vi "LEP_RV_StartLaunch.vi"(8 "error in (no error)":errorcluster) -> (0 "error out":errorcluster)   [LabVIEW 2011]
doc: "Download and execute built VxWorks downloadable module and attach the LabVIEW Embedded debuger."
uses:
  LEP_RV_Commands.ctl
  LEP_RV_Config.ctl
  <vilib>/Platform/EmbProject/utilities/Emb_Utility_AppAction.ctl
  <vilib>/LabVIEW Targets/Embedded/ASWServer/MPU_ASWServer_GeneralIcons.ctl
  <vilib>/LabVIEW Targets/Embedded/ASWServer/MPU_ASWServer_GeneralCtrls.ctl
  LEP_RV_LaunchGlobals.vi
  <vilib>/Platform/EmbProject/Plugins/utilities/LEP_Utilities_GetInfoGlobals.vi
  <vilib>/Instr/_visa.llb/VISA Configure Serial Port (Instr).vi
panel:
  in  "Client installed":bool
  in  "Remember password":bool
  in  "Password":string
  in  "User name":string
  in  "Compiler server name":string
  in  "Connect to a network compile server":bool
  in  "buildSpec ID":string
  in  "error string":string
  in  "Error Indicator":bool[](array[boolean])
  in  "Node ID List":i32[](array[numeric])
  in  "Message List":string[][](array[string])
  in  "Active File Count":i32
  in  "embeddedSessionID":u32
  in  "subtarget":string
  in  "path":path
  in  "preallocate UI Enabled":bool
  in  "target display name":string
  in  "SourceFiles":path[](array[path])
  in  "ExternalFiles":path[](array[path])
  in  "ProjectPath":path
  in  "display name":string
  in  "typeID":string
  in  "debug occurrence":refnum<k4>
  in  "Item ID":string
  in  "Root ID":string
  in  "target ID":u32
  in  "build ID":u32
  in  "MaxElements":u32
  in  "DebugSerialPort":string
  in  "DebugSerialBaud":u32
  in  "Context":refnum<vi>
  in  "UpdateClusters":u32
  in  "UpdateArrays":u32
  in  "Update":u32
  in  "BreakpointsConfig":cluster{"Clear on Start":bool}
  in  "File List":path[](array[path])
  in  "action":T1
  in  "Config":T2={"Enable debugging"=FALSE, "Debug Options"=0, "Use stack variables"=FALSE, "Generate serial only"=FALSE, "Generate guard code"=FALSE, "Generate Integer Only"=FALSE, "Generate C Function Calls"=TRUE, "ExpressionFolding"=TRUE, "Constant Allocation"=0, "Constant Deallocation"=0, "Build Specification ID"="", "Preprocessor symbols (define)"="", "Compiler Flags"="", "Linker Flags"="", "Mode"=1, "Optimization"=2, "Optimize for time"=FALSE, "Enable cross-module optimization"=FALSE, "Include paths"=[], "Optimize heap size"=TRUE, "Use MicroLib"=FALSE, "Debug Mode"=2, "Enable profile information"=FALSE, "Host name"="board", "Use DHCP"=TRUE, "IP address"="0.0.0.0", "Subnet mask"="", "Gateway"="0.0.0.0", "Primary DNS"="0.0.0.0", "Secondary DNS"="0.0.0.0", "MAC in target memory"=TRUE, "MAC address"="", "Console output"=1, "Target serial port"=1} {"Constant Deallocation" items=["Out of Scope", "VI End", "Application End"]; "Constant Allocation" items=["First Use", "Containing Loop", "VI Initialization", "Application Initialization"]; "Target serial port" items=["0", "1", "2", "3"]; "Console output" items=["Processor status window", "Serial port"]; "Optimization" items=["Level 0 (-O0)", "Level 1 (-O1)", "Level 2 (-O2)", "Level 3 (-O3)"]; "Mode" items=["ARM-Mode", "Thumb-Mode"]; "Debug Options" items=["Use ULINK Debugger", "Use Simulator"]; "Debug Mode" items=["Instrumented (serial port)", "Instrumented (TCP/IP)", "Non-instrumented (JTAG/USB)"]}
  in  "TopLevelVI":path
  in  "UV Project File":path
  in  "Target Name":string
  in  "Build Path":path
  in  "Commands":T3
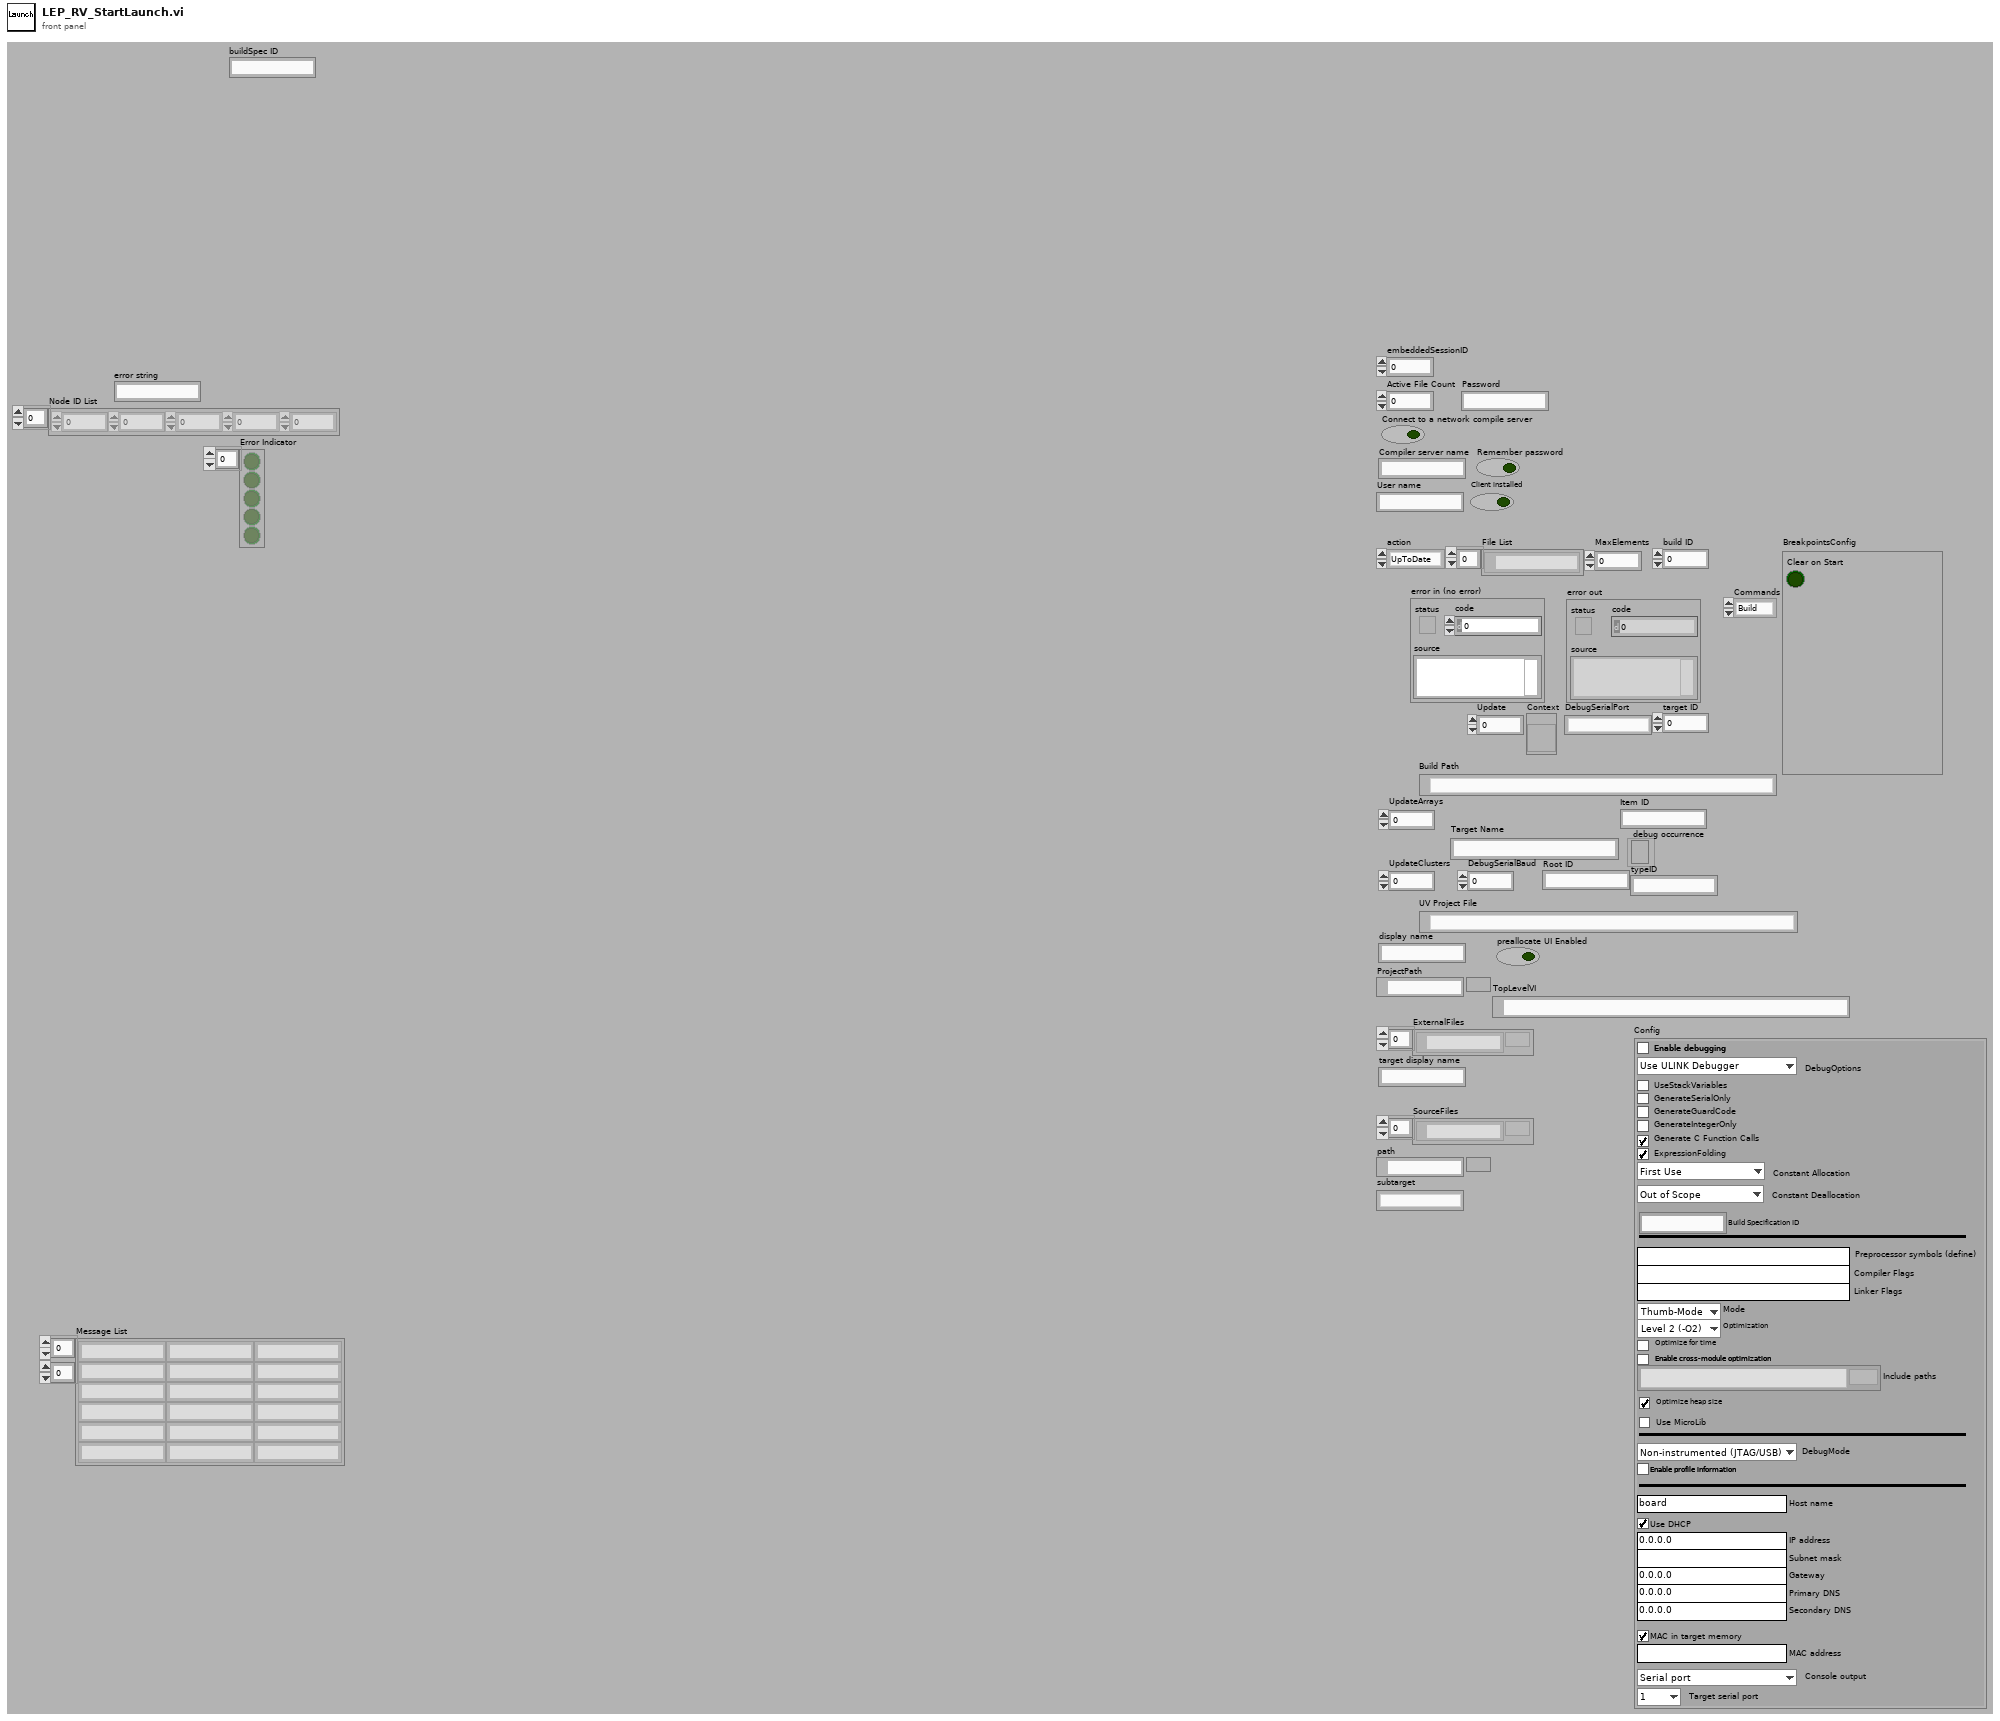
[diagram p1: front panel]
types:
  T1 = typedef "Emb_Utility_AppAction.ctl" = enum16{"UpToDate", "Build", "Cancel", "Error"}
  T2 = typedef "LEP_RV_Config.ctl" = cluster{"Enable debugging":bool, "Debug Options":u16, "Use stack variables":bool, "Generate serial only":bool, "Generate guard code":bool, "Generate Integer Only":bool, "Generate C Function Calls":bool, "ExpressionFolding":bool, "Constant Allocation":u16, "Constant Deallocation":u16, "Build Specification ID":string, "Preprocessor symbols (define)":string, "Compiler Flags":string, "Linker Flags":string, "Mode":u16, "Optimization":u16, "Optimize for time":bool, "Enable cross-module optimization":bool, "Include paths":path[], "Optimize heap size":bool, "Use MicroLib":bool, "Debug Mode":u16, "Enable profile information":bool, "Host name":string, "Use DHCP":bool, "IP address":string, "Subnet mask":string, "Gateway":string, "Primary DNS":string, "Secondary DNS":string, "MAC in target memory":bool, "MAC address":string, "Console output":u16, "Target serial port":u16}
  T3 = typedef "LEP_RV_Commands.ctl" = enum16{"Build", "Rebuild", "Run", "Debug", "Profile"}
  T4 = typedef "MPU_ASWServer_GeneralIcons.ctl" = enum16{"Complete", "Disconnected", "Error", "Initializing", "Ready", "Running", "Stopped", "Unknown", "No Change"}
  T5 = typedef "MPU_ASWServer_GeneralCtrls.ctl" = enum16{"Build Status", "Download Status", "Target Name", "Target Type", "Application Name"}
  T6 = enum16{"Build Successful", "Build Failed", "Build Cancelled"}
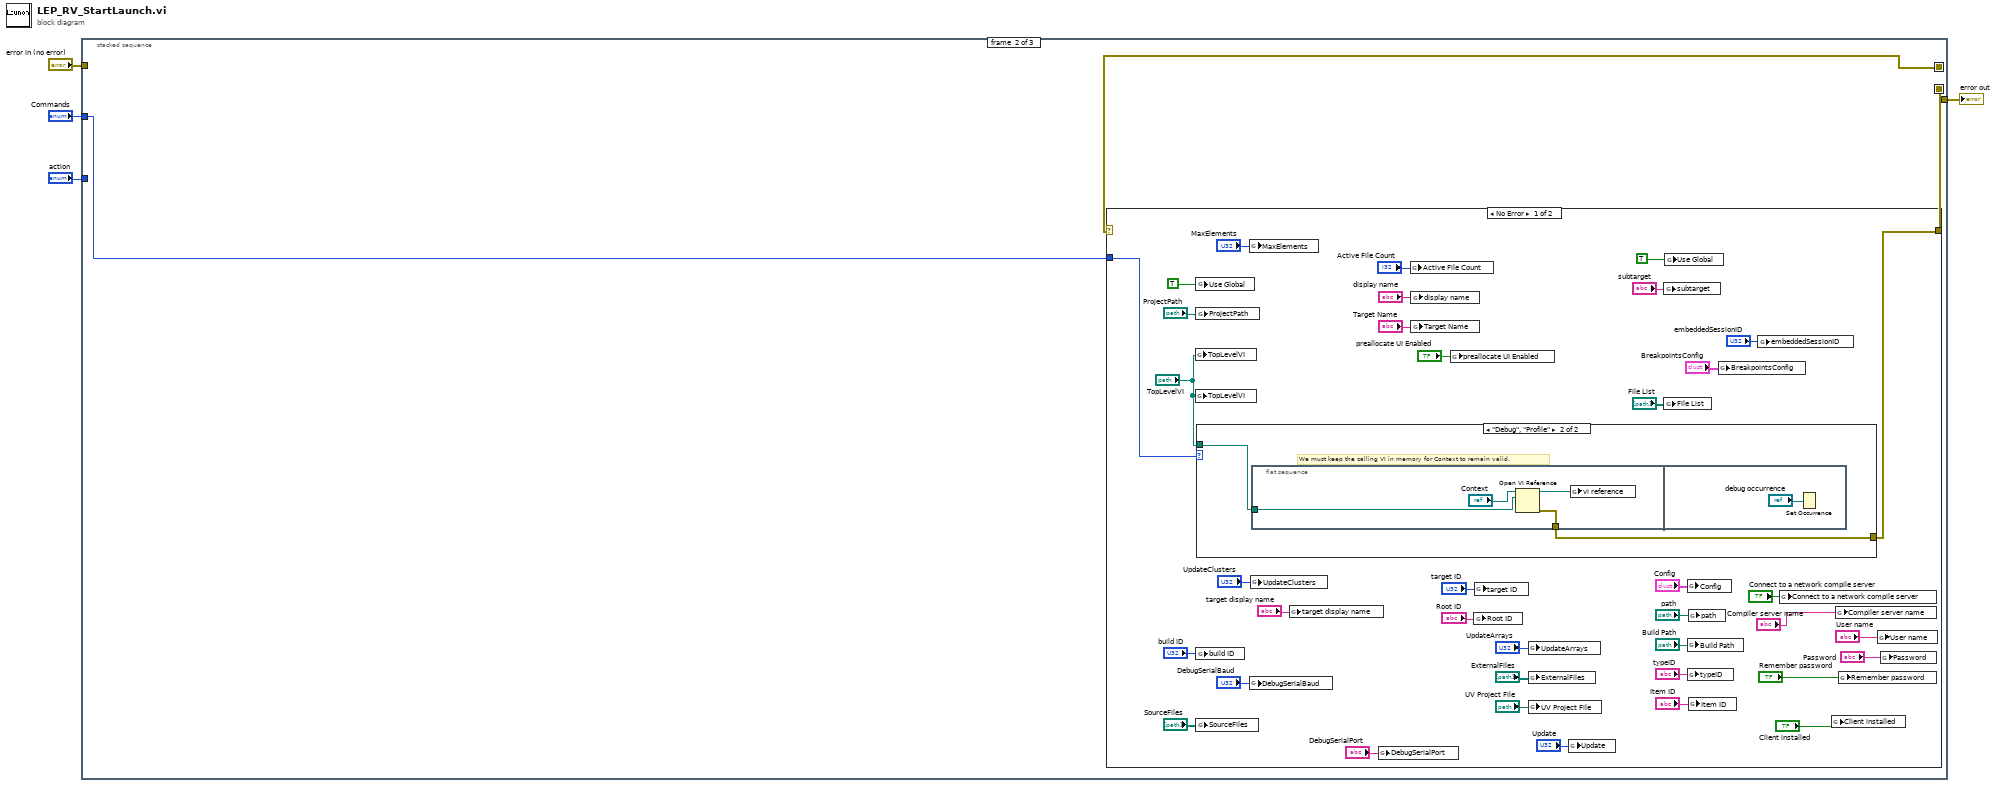
[diagram p0: block diagram]
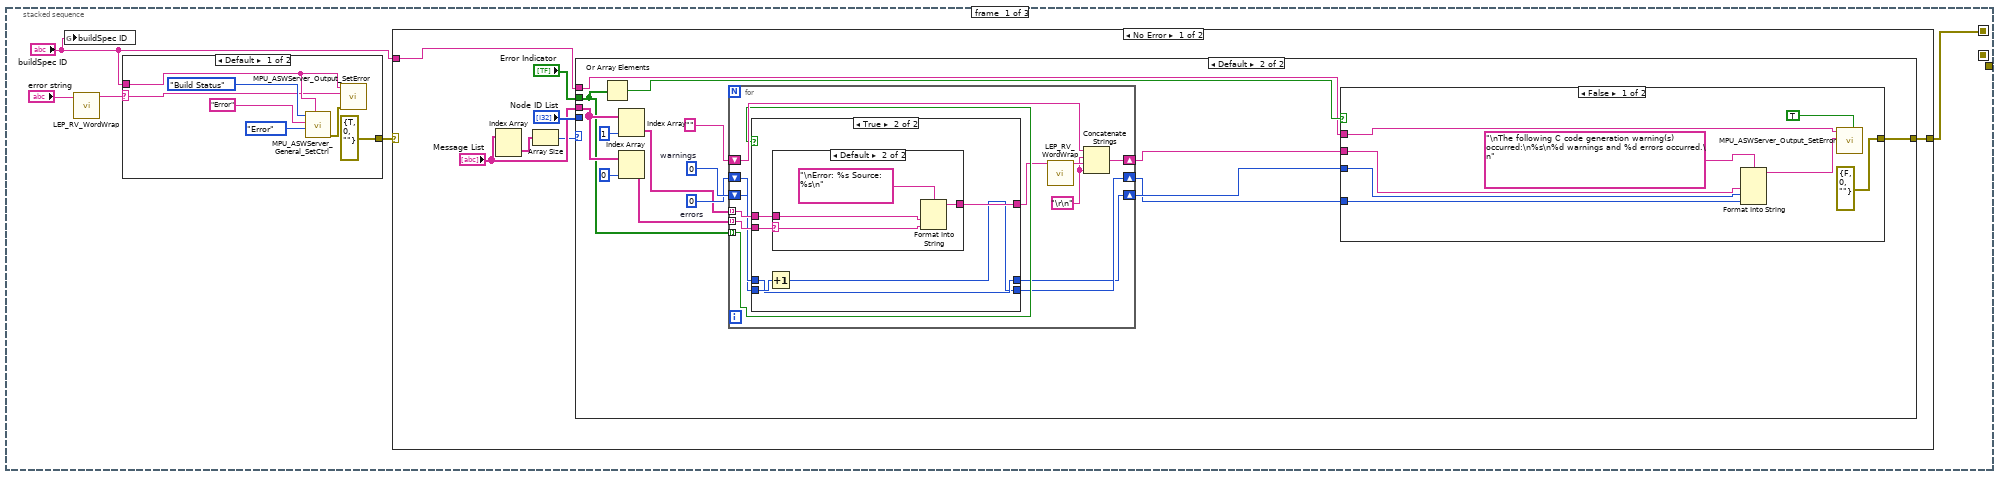
[diagram p2: hidden frame]
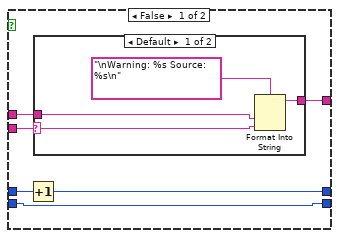
[diagram p4: hidden frame]
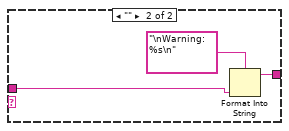
[diagram p5: hidden frame]
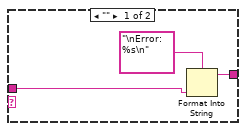
[diagram p6: hidden frame]
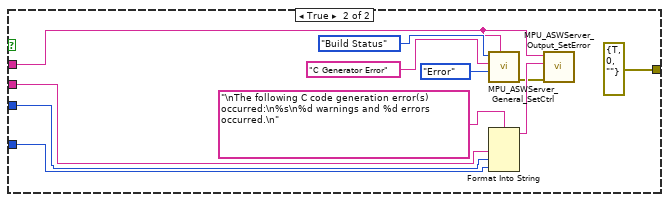
[diagram p7: hidden frame]
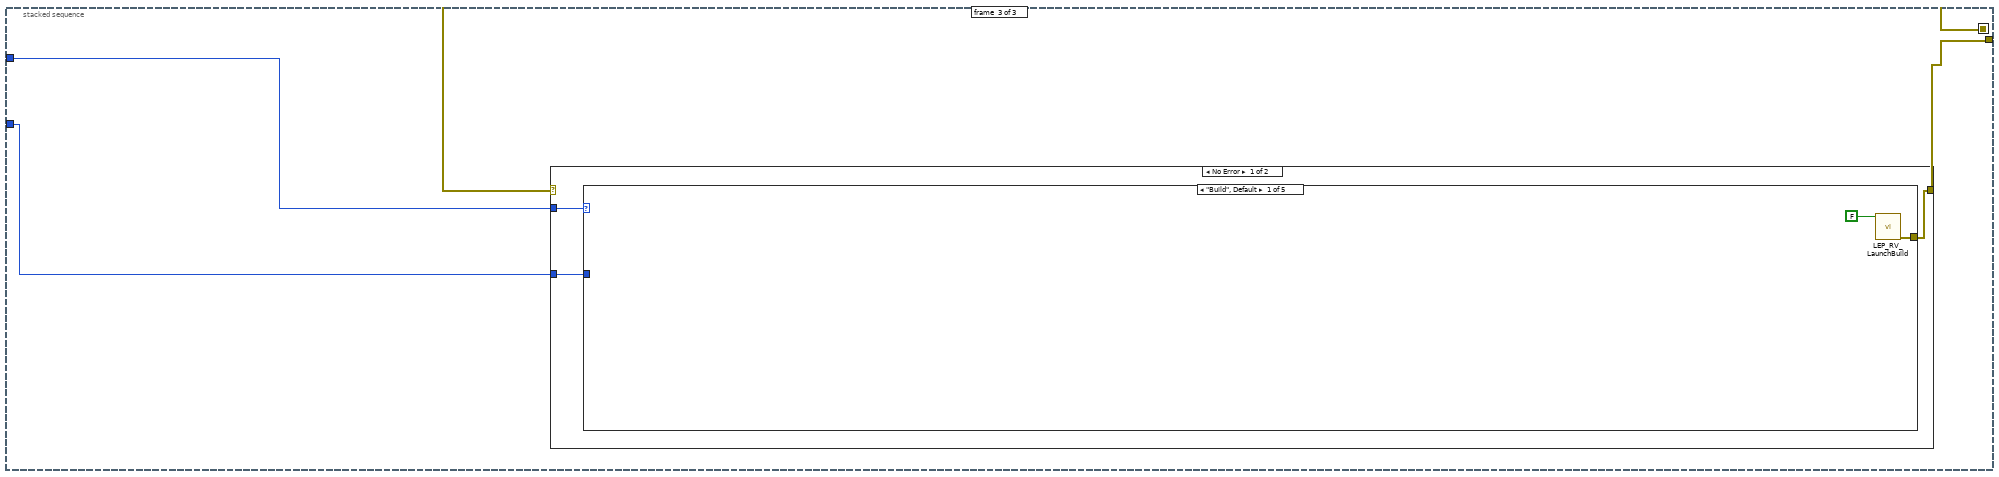
[diagram p12: hidden frame]
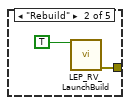
[diagram p13: hidden frame]
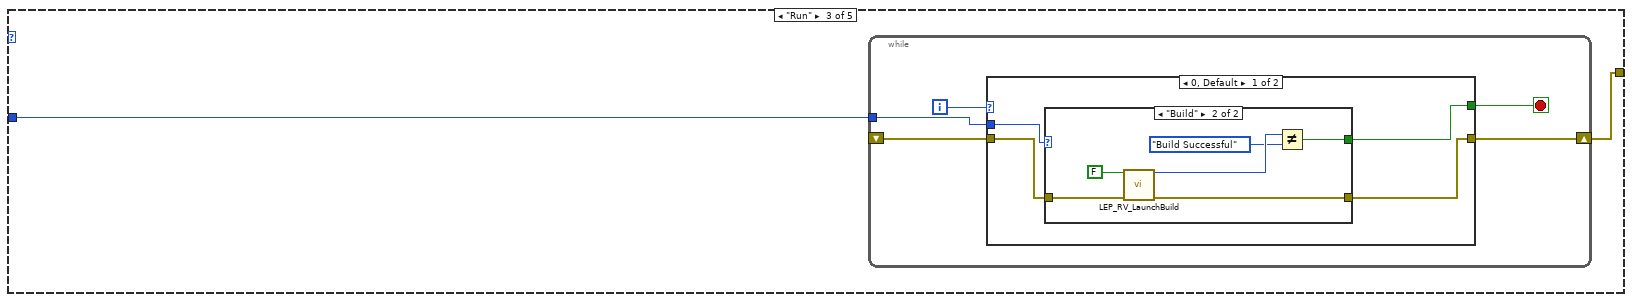
[diagram p14: hidden frame]
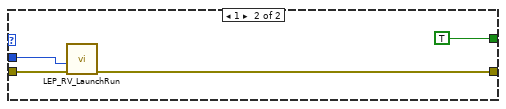
[diagram p16: hidden frame]
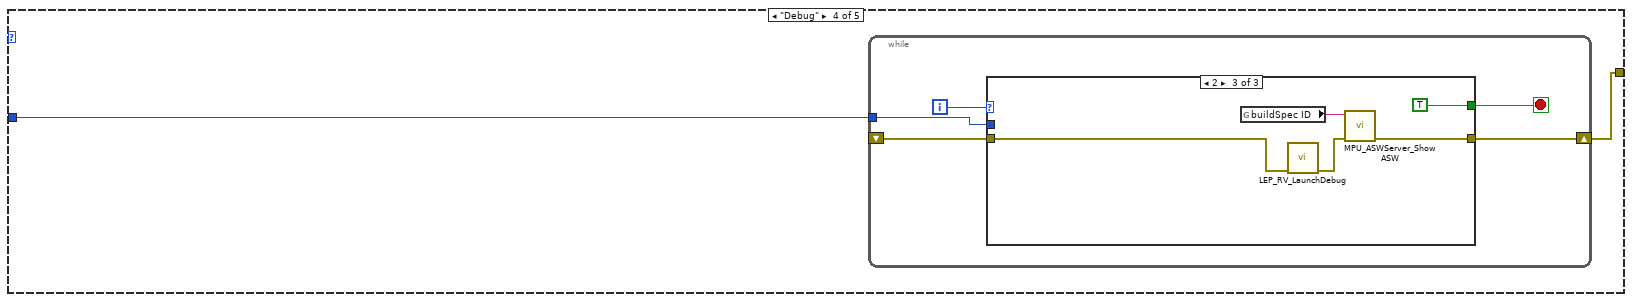
[diagram p17: hidden frame]
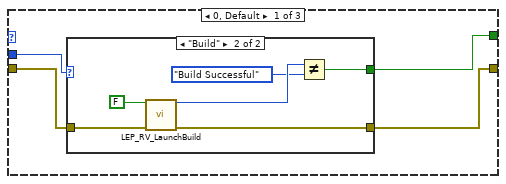
[diagram p18: hidden frame]
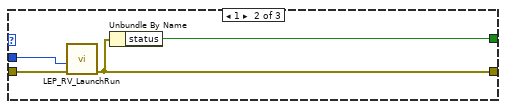
[diagram p20: hidden frame]
diagram:
  n1 = stacked-sequence {
    seq-local: [_ w98 _] -> [_ _ w146]
    seq-local: [w8 _ _] -> [_ w97 _]
    tunnel: "error in (no error)" -> [_ _ _]
    tunnel: [_ _ w149] -> w3
    tunnel: "Commands" -> [_ w99 w148]
    tunnel: "action" -> [_ _ w147]
    frame #0 {
      n2 = global write "LEP_RV_LaunchGlobals.vi" "buildSpec ID"("buildSpec ID") -> ()
      n3 = call "LEP_RV_WordWrap.vi"("input string"="error string") -> ("output string"=w5:string)  [unwired: 10 in]
      n4 = case shown="Default" w5 {
        selector: w5 -> [w92 _]
        tunnel: "buildSpec ID" -> [w96 _]
        tunnel: [errorcluster {"status"=TRUE, "code"=0, "source"=""} ("error out") _] -> w7
        frame Default {
          n5 = call <vilib>:"MPU_ASWServer_General_SetCtrl.vi"("buildSpec ID"=w96, "icon"=MPU_ASWServer_GeneralIcons."Error", "value"="Error", "control"=MPU_ASWServer_GeneralCtrls."Build Status") -> ("error out"=w91:errorcluster)  [unwired: 5 in, 2 out]
          n6 = call <vilib>:"MPU_ASWServer_Output_SetError.vi"("error in"=w91, "error str"=w92, "buildSpec ID"=w96) -> ()  [unwired: 2 in, 5 out]
        }
        frame "", "CGenErr" {
        }
      }
      n7 = case shown="No Error" w7 {
        selector: w7 -> [_ w89]
        tunnel: "buildSpec ID" -> [w14 _]
        tunnel: [w10 w89] -> w8
        frame No Error {
          n8 = Index Array(array="Message List") -> (element=w12:string[])  [unwired: 2 in]
          n9 = Array Size(array=w12) -> (size(s)=w11:i32)
          n10 = case shown="Default" w11 {
            tunnel: "Message List" -> [_ w23]
            tunnel: "Error Indicator" -> [_ w22]
            tunnel: "Node ID List" -> [_ _]
            tunnel: w14 -> [_ w21]
            tunnel: [_ w20] -> w10
            frame 0 {
            }
            frame Default {
              w29 = u32 0  # warnings
              w28 = u32 0  # errors
              n11 = Or Array Elements(Boolean array=w22) -> (logical OR=w24:bool)
              n12 = Index Array(array=w23, index (col)=1 ("index (row)")) -> (element=w26:string[])  [unwired: 1 in]
              n13 = Index Array(array=w23, index (col)=0 ("index (row)")) -> (element=w27:string[])  [unwired: 1 in]
              n14 = for {
                shift-right: [w42] -> w17
                shift-left: "" -> [w43]
                tunnel: w26 -> [w41] mode=indexing
                tunnel: w27 -> [w40] mode=indexing
                tunnel: w22 -> [w39] mode=indexing
                shift-right: [w36] -> w30
                shift-left: w28 -> [w37]
                shift-right: [w35] -> w31
                shift-left: w29 -> [w38]
                w32 = "\r\n"
                n15 = case shown="True" w39 {
                  tunnel: [w48 w62] -> w34
                  tunnel: w41 -> [w49 w61]
                  tunnel: w40 -> [w44 w57]
                  tunnel: w38 -> [w46 w59]
                  tunnel: w37 -> [w47 w60]
                  tunnel: [w47 w58] -> w36
                  tunnel: [w45 w59] -> w35
                  frame False {
                    n16 = Increment(x=w46) -> (x+1=w45:u32)
                    n17 = case shown="Default" w44 {
                      selector: w44 -> [w52 _]
                      tunnel: w49 -> [w51 w55]
                      tunnel: [w50 w54] -> w48
                      frame Default {
                        n18 = Format Into String(format string="\nWarning: %s Source: %s\n", w51, w52) -> (resulting string=w50:string)  [unwired: 2 in, 1 out]
                      }
                      frame "" {
                        n19 = Format Into String(format string="\nWarning: %s\n", w55) -> (resulting string=w54:string)  [unwired: 2 in, 1 out]
                      }
                    }
                  }
                  frame True {
                    n20 = Increment(x=w60) -> (x+1=w58:u32)
                    n21 = case shown="Default" w57 {
                      selector: w57 -> [_ w66]
                      tunnel: [w64 w68] -> w62
                      tunnel: w61 -> [w63 w67]
                      frame "" {
                        n22 = Format Into String(format string="\nError: %s\n", w63) -> (resulting string=w64:string)  [unwired: 2 in, 1 out]
                      }
                      frame Default {
                        n23 = Format Into String(format string="\nError: %s Source: %s\n", w67, w66) -> (resulting string=w68:string)  [unwired: 2 in, 1 out]
                      }
                    }
                  }
                }
                n24 = call "LEP_RV_WordWrap.vi"("input string"=w34) -> ("output string"=w33:string)  [unwired: 10 in]
                n25 = Concatenate Strings(w43, w32, w33, w32) -> (w42:string)
              }
              n26 = case shown="False" w24 {
                tunnel: w21 -> [w72 w81]
                tunnel: w30 -> [w73 w79]
                tunnel: w31 -> [w74 w78]
                tunnel: w17 -> [w75 w87]
                tunnel: [errorcluster {"status"=FALSE, "code"=0, "source"=""} ("error out") errorcluster {"status"=TRUE, "code"=0, "source"=""} ("error out")] -> w20
                frame False {
                  n27 = Format Into String(format string="\nThe following C code generation warning(s) occurred:\n%s\n%d warnings and %d errors occurred.\n", w75, w74, w73) -> (resulting string=w71:string)  [unwired: 2 in, 1 out]
                  n28 = call <vilib>:"MPU_ASWServer_Output_SetError.vi"("warning only (F)"=TRUE ("warning only"), "error str"=w71, "buildSpec ID"=w72) -> ()  [unwired: 2 in, 5 out]
                }
                frame True {
                  n29 = call <vilib>:"MPU_ASWServer_General_SetCtrl.vi"("buildSpec ID"=w81, "icon"=MPU_ASWServer_GeneralIcons."Error", "value"="C Generator Error", "control"=MPU_ASWServer_GeneralCtrls."Build Status") -> ("error out"=w82:errorcluster)  [unwired: 5 in, 2 out]
                  n30 = Format Into String(format string="\nThe following C code generation error(s) occurred:\n%s\n%d warnings and %d errors occurred.\n", w87, w78, w79) -> (resulting string=w86:string)  [unwired: 2 in, 1 out]
                  n31 = call <vilib>:"MPU_ASWServer_Output_SetError.vi"("error in"=w82, "error str"=w86, "buildSpec ID"=w81) -> ()  [unwired: 2 in, 5 out]
                }
              }
            }
          }
        }
        frame Error {
        }
      }
    }
    frame #1 {
      n32 = case shown="No Error" w97 {
        selector: w97 -> [_ w145]
        tunnel: w99 -> [w137 _]
        tunnel: [w136 w145] -> w98
        frame No Error {
          n33 = global write "LEP_RV_LaunchGlobals.vi" "TopLevelVI"("TopLevelVI") -> ()
          n34 = global write "LEP_Utilities_GetInfoGlobals.vi" "TopLevelVI"("TopLevelVI") -> ()
          n35 = global write "LEP_Utilities_GetInfoGlobals.vi" "Use Global"(TRUE ("Use Global")) -> ()
          n36 = global write "LEP_Utilities_GetInfoGlobals.vi" "ProjectPath"("ProjectPath") -> ()
          n37 = global write "LEP_RV_LaunchGlobals.vi" "build ID"("build ID") -> ()
          n38 = global write "LEP_Utilities_GetInfoGlobals.vi" "SourceFiles"("SourceFiles") -> ()
          n39 = case shown="\"Debug\", \"Profile\"" w137 {
            tunnel: "TopLevelVI" -> [_ w139]
            tunnel: [_ w138] -> w136
            frame Default {
            }
            frame "Debug", "Profile" {
              # "We must keep the calling VI in memory for Context to remain valid."
              n40 = flat-sequence {
                tunnel: w139 -> [w143]
                tunnel: [w140] -> w138
                frame #0 {
                  n41 = Open VI Reference(application reference (local)="Context", vi path=w143) -> (vi reference=w142:refnum<vi>, error out=w140:errorcluster)  [unwired: 4 in]
                  n42 = global write "LEP_RV_LaunchGlobals.vi" "vi reference"(w142) -> ()
                }
                frame #1 {
                  n43 = Set Occurrence("debug occurrence") -> ()
                }
              }
            }
          }
          n44 = global write "LEP_RV_LaunchGlobals.vi" "MaxElements"("MaxElements") -> ()
          n45 = global write "LEP_RV_LaunchGlobals.vi" "DebugSerialBaud"("DebugSerialBaud") -> ()
          n46 = global write "LEP_RV_LaunchGlobals.vi" "UpdateClusters"("UpdateClusters") -> ()
          n47 = global write "LEP_Utilities_GetInfoGlobals.vi" "target display name"("target display name") -> ()
          n48 = global write "LEP_RV_LaunchGlobals.vi" "DebugSerialPort"("DebugSerialPort") -> ()
          n49 = global write "LEP_RV_LaunchGlobals.vi" "Active File Count"("Active File Count") -> ()
          n50 = global write "LEP_Utilities_GetInfoGlobals.vi" "display name"("display name") -> ()
          n51 = global write "LEP_RV_LaunchGlobals.vi" "Target Name"("Target Name") -> ()
          n52 = global write "LEP_Utilities_GetInfoGlobals.vi" "preallocate UI Enabled"("preallocate UI Enabled") -> ()
          n53 = global write "LEP_RV_LaunchGlobals.vi" "Root ID"("Root ID") -> ()
          n54 = global write "LEP_RV_LaunchGlobals.vi" "target ID"("target ID") -> ()
          n55 = global write "LEP_RV_LaunchGlobals.vi" "UpdateArrays"("UpdateArrays") -> ()
          n56 = global write "LEP_Utilities_GetInfoGlobals.vi" "ExternalFiles"("ExternalFiles") -> ()
          n57 = global write "LEP_RV_LaunchGlobals.vi" "UV Project File"("UV Project File") -> ()
          n58 = global write "LEP_RV_LaunchGlobals.vi" "Update"("Update") -> ()
          n59 = global write "LEP_Utilities_GetInfoGlobals.vi" "subtarget"("subtarget") -> ()
          n60 = global write "LEP_RV_LaunchGlobals.vi" "File List"("File List") -> ()
          n61 = global write "LEP_RV_LaunchGlobals.vi" "Use Global"(TRUE ("Use Global")) -> ()
          n62 = global write "LEP_RV_LaunchGlobals.vi" "Config"("Config") -> ()
          n63 = global write "LEP_RV_LaunchGlobals.vi" "Build Path"("Build Path") -> ()
          n64 = global write "LEP_Utilities_GetInfoGlobals.vi" "typeID"("typeID") -> ()
          n65 = global write "LEP_Utilities_GetInfoGlobals.vi" "path"("path") -> ()
          n66 = global write "LEP_RV_LaunchGlobals.vi" "Item ID"("Item ID") -> ()
          n67 = global write "LEP_RV_LaunchGlobals.vi" "BreakpointsConfig"("BreakpointsConfig") -> ()
          n68 = global write "LEP_RV_LaunchGlobals.vi" "embeddedSessionID"("embeddedSessionID") -> ()
          n69 = global write "LEP_RV_LaunchGlobals.vi" "Connect to a network compile server"("Connect to a network compile server") -> ()
          n70 = global write "LEP_RV_LaunchGlobals.vi" "Client installed"("Client installed") -> ()
          n71 = global write "LEP_RV_LaunchGlobals.vi" "Compiler server name"("Compiler server name") -> ()
          n72 = global write "LEP_RV_LaunchGlobals.vi" "Remember password"("Remember password") -> ()
          n73 = global write "LEP_RV_LaunchGlobals.vi" "User name"("User name") -> ()
          n74 = global write "LEP_RV_LaunchGlobals.vi" "Password"("Password") -> ()
        }
        frame Error {
        }
      }
    }
    frame #2 {
      n75 = case shown="No Error" w146 {
        selector: w146 -> [_ w259]
        tunnel: [w152 w259] -> w149
        tunnel: w148 -> [w151 _]
        tunnel: w147 -> [w150 _]
        frame No Error {
          n76 = case shown="\"Build\", Default" w151 {
            tunnel: [w153 w155 w157 w179 w206] -> w152
            tunnel: w150 -> [_ _ w158 w180 w207]
            frame "Build", Default {
              n77 = call "LEP_RV_LaunchBuild.vi"("Rebuild"=FALSE) -> ("error out"=w153:errorcluster)  [unwired: 13 in, 1 out]
            }
            frame "Rebuild" {
              n78 = call "LEP_RV_LaunchBuild.vi"("Rebuild"=TRUE) -> ("error out"=w155:errorcluster)  [unwired: 13 in, 1 out]
            }
            frame "Run" {
              n79 = while {
                tunnel: w158 -> [w161]
                shift-right: [w159] -> w157
                shift-left: _ -> [w160]
                i -> [w163]
                stop <- w162 stop-if-true
                n80 = case shown="0, Default" w163 {
                  tunnel: [w166 TRUE] -> w162
                  tunnel: w161 -> [w167 w177]
                  tunnel: w160 -> [w165 w176]
                  tunnel: [w164 w175] -> w159
                  frame 0, Default {
                    n81 = case shown="\"Build\"" w167 {
                      tunnel: [_ w171] -> w166
                      tunnel: w165 -> [w168 w170]
                      tunnel: [w168 w169] -> w164
                      frame "UpToDate", Default {
                      }
                      frame "Build" {
                        n82 = call "LEP_RV_LaunchBuild.vi"("Rebuild"=FALSE, "error in (no error)"=w170) -> ("Build Result"=w173:T6, "error out"=w169:errorcluster)  [unwired: 12 in]
                        n83 = Not Equal?(x=w173, y=T6."Build Successful") -> (x != y?=w171:bool)
                      }
                    }
                  }
                  frame 1 {
                    n84 = call "LEP_RV_LaunchRun.vi"("error in (no error)"=w176, "action"=w177) -> ("error out"=w175:errorcluster)  [unwired: 9 in]
                  }
                }
              }
            }
            frame "Debug" {
              n85 = while {
                tunnel: w180 -> [w184]
                shift-right: [w181] -> w179
                shift-left: _ -> [w182]
                i -> [w185]
                stop <- w183 stop-if-true
                n86 = case shown="2" w185 {
                  tunnel: w184 -> [w189 w200 _]
                  tunnel: [w188 w199 TRUE ("status")] -> w183
                  tunnel: w182 -> [w187 w198 w204]
                  tunnel: [w186 w197 w201] -> w181
                  frame 0, Default {
                    n87 = case shown="\"Build\"" w189 {
                      tunnel: [_ w193] -> w188
                      tunnel: w187 -> [w190 w192]
                      tunnel: [w190 w191] -> w186
                      frame "UpToDate", Default {
                      }
                      frame "Build" {
                        n88 = call "LEP_RV_LaunchBuild.vi"("Rebuild"=FALSE, "error in (no error)"=w192) -> ("Build Result"=w195:T6, "error out"=w191:errorcluster)  [unwired: 12 in]
                        n89 = Not Equal?(x=w195, y=T6."Build Successful") -> (x != y?=w193:bool)
                      }
                    }
                  }
                  frame 1 {
                    n90 = call "LEP_RV_LaunchRun.vi"("error in (no error)"=w198, "action"=w200) -> ("error out"=w197:errorcluster)  [unwired: 9 in]
                    n91 = Unbundle By Name(w197) -> ("status"=w199:bool)
                  }
                  frame 2 {
                    n92 = global read "LEP_RV_LaunchGlobals.vi" "buildSpec ID"() -> (w203:string)
                    n93 = call "LEP_RV_LaunchDebug.vi"("error in (no error)"=w204) -> ("error out"=w202:errorcluster)  [unwired: 10 in]
                    n94 = call <vilib>:"MPU_ASWServer_Show ASW.vi"("error in (no error)"=w202, "buildSpec ID"=w203) -> ("error out"=w201:errorcluster)  [unwired: 8 in, 1 out]
                  }
                }
              }
            }
            frame "Profile" {
              n95 = while {
                tunnel: w207 -> [w213]
                shift-right: [w210] -> w206
                shift-left: _ -> [w211]
                shift-right: [w209] -> _
                shift-left: _ -> [w208]
                i -> [w214]
                stop <- w212 stop-if-true
                n96 = case shown="4" w214 {
                  tunnel: w213 -> [w218 _ w248 _ _]
                  tunnel: [w217 w230 w247 w251 TRUE ("status")] -> w212
                  tunnel: w211 -> [w216 w226 w246 w252 w257]
                  tunnel: [w215 w231 w245 w249 w253] -> w210
                  tunnel: [_ w232 w244 w250 _] -> w209
                  tunnel: w208 -> [_ _ w244 w250 w256]
                  frame 0, Default {
                    n97 = case shown="\"UpToDate\", Default" w218 {
                      tunnel: [_ w222] -> w217
                      tunnel: w216 -> [w219 w221]
                      tunnel: [w219 w220] -> w215
                      frame "UpToDate", Default {
                      }
                      frame "Build" {
                        n98 = call "LEP_RV_LaunchBuild.vi"("Rebuild"=FALSE, "error in (no error)"=w221) -> ("Build Result"=w224:T6, "error out"=w220:errorcluster)  [unwired: 12 in]
                        n99 = Not Equal?(x=w224, y=T6."Build Successful") -> (x != y?=w222:bool)
                      }
                    }
                  }
                  frame 1 {
                    n100 = global read "LEP_RV_LaunchGlobals.vi" "DebugSerialPort"() -> (w228:string)
                    n101 = case shown="\"\"" w228 {
                      selector: w228 -> [w242 _]
                      tunnel: [w242 "COM1" ("t")] -> w233
                      frame Default {
                      }
                      frame "" {
                      }
                    }
                    n102 = global read "LEP_RV_LaunchGlobals.vi" "DebugSerialBaud"() -> (w227:u32)
                    n103 = call-poly "VISA Configure Serial Port"("VISA resource name"=w233, "timeout (10sec)"=u32 250, "termination char\n(0xA = '\\n' = LF)"=u8 13 ("termination char\n(0xA = '\\n' = LF)"), "Enable Termination\nChar (T)"=TRUE ("Enable Termination\nChar (T)"), "baud rate (9600)"=w227, "error in (no error)"=w226) -> ("VISA resource name out"=w232:refnum<visa-resource-name>, "error out"=w231:errorcluster)  [unwired: 3 in, 5 out]
                    n104 = Unbundle By Name(w231) -> ("code"=w229:i32, "status"=w230:bool)
                    n105 = case shown="Default" w229 {
                      frame Default {
                      }
                      frame -1073807246 {
                        n106 = call <vilib>:"Three Button Dialog.vi"("Window Title (\"\")"="Profiling Error" ("Window Title (\"\")"), "Right Button Text (\"Cancel\")"="" ("Right Button Text (\"Cancel\")"), "Center Button Text (\"No\")"="OK" ("Center Button Text (\"No\")"), "Left Button Text (\"Yes\")"="" ("Left Button Text (\"Yes\")"), "message"="An error occurred while opening the serial port. \nPlease close any programs that are using the serial port.") -> ()  [unwired: 6 in, 1 out]
                      }
                    }
                  }
                  frame 2 {
                    n107 = call "LEP_RV_LaunchRun.vi"("error in (no error)"=w246, "action"=w248) -> ("error out"=w245:errorcluster)  [unwired: 9 in]
                    n108 = Unbundle By Name(w245) -> ("status"=w247:bool)
                  }
                  frame 3 {
                    n109 = call "LEP_RV_LaunchDebug.vi"("error in (no error)"=w252) -> ("error out"=w249:errorcluster)  [unwired: 10 in]
                    n110 = Unbundle By Name(w249) -> ("status"=w251:bool)
                  }
                  frame 4 {
                    n111 = global read "LEP_RV_LaunchGlobals.vi" "buildSpec ID"() -> (w255:string)
                    n112 = call "LEP_RV_LaunchProfile.vi"("error in (no error)"=w257, "VISA resource name"=w256) -> ("error out"=w254:errorcluster)  [unwired: 9 in]
                    n113 = call <vilib>:"MPU_ASWServer_Show ASW.vi"("error in (no error)"=w254, "buildSpec ID"=w255) -> ("error out"=w253:errorcluster)  [unwired: 8 in, 1 out]
                  }
                }
              }
            }
          }
        }
        frame Error {
        }
      }
    }
  }
  "error out" <- w3
